vi "Motion_Profiling.vi"() -> ()   [LabVIEW 2015]
uses:
  <vilib>/Rock Robotics/WPI/Utilities/WPI_GetSetVariantRefNum.vi
panel:
  in  "Max Speed":dbl=120.0 format="%#_13g"
  in  "Max Accel":dbl=80.0 format="%#_13g"
  in  "Max Jerk":dbl=80.0 format="%#_13g"
  in  "forward":bool=TRUE
  in  "DistanceR (in)":dbl=180.0
  in  "DistanceL (in)":dbl=180.0
  in  "Auto Control":bool=TRUE
  in  "Constants":T1={"kV"=0.009, "kA"=0.0, "PV"=0.0, "PP"=0.0, "DV"=0.0}
  out "Position Chart":cluster{"pos":dbl, "pos":dbl, "pos":dbl}(graph)
  in  "Duty Cycle":dbl(slide)=0.015603286203016431 scale=-1.0..1.0
  out "Velocity Chart":cluster{"vel":dbl, dbl, "vel":dbl}(graph)
  in  "Chart Slowing":u32(knob)=4 scale=1.0..10.0
  # "Remember to make default!"
  # "backward"
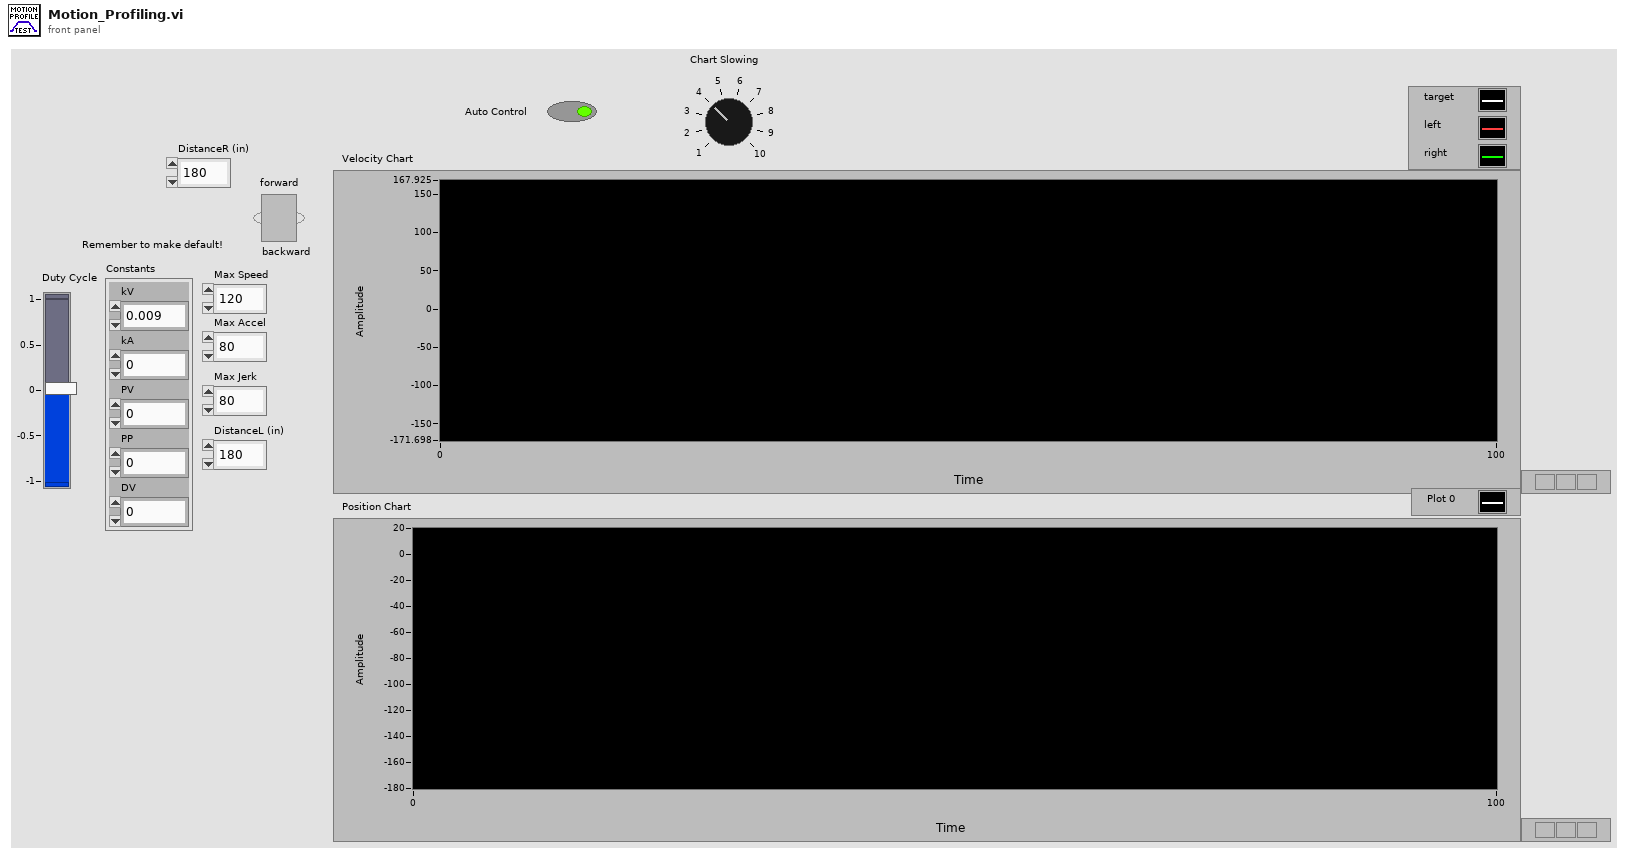
[diagram p1: front panel]
types:
  T1 = cluster{"kV":dbl, "kA":dbl, "PV":dbl, "PP":dbl, "DV":dbl}
  T2 = cluster{"Positions":dbl[], "Velocities":dbl[], "Accelerations":dbl[]}
  T3 = typedef "WPI_PotentiometerDevRef.ctl" = cluster{"DevStatus":errorcluster, "Analog Channel":T4, "Invert Output":bool}
  T4 = typedef "FPGA_AIChannel.ctl" = enum8{"AI 0", "AI 1", "AI 2", "AI 3", "AI MXP 0", "AI MXP 1", "AI MXP 2", "AI MXP 3", "Invalid"}
  T5 = typedef "WPI_RobotDriveDevRef.ctl" = cluster{"DevStatus":errorcluster, "Motors[]":T6[], "Square Inputs":bool, "Max Output":dbl}
  T6 = typedef "WPI_MotorControlDeviceRef.ctl" = cluster{"DeviceStatus":errorcluster, "Type":T7, "PWM":cluster{"PWM Channel":T8, "DeadBand":T9}, "CAN":cluster{"Device Number":u8, "Control Mode":T10, "Semaphore":T11, "Max Vout":dbl, "TalonSRX Control Mode":T12}, "Invert":bool}
  T7 = typedef "WPI_MotorControlType.ctl" = enum16{"PWM", "CAN", "CANTalonSRX"}
  T8 = typedef "FPGA_DIOPWMChannel.ctl" = enum8{"PWM 0", "PWM 1", "PWM 2", "PWM 3", "PWM 4", "PWM 5", "PWM 6", "PWM 7", "PWM 8", "PWM 9", "PWM MXP 0", "PWM MXP 1", "PWM MXP 2", "PWM MXP 3", "PWM MXP 4", "PWM MXP 5", "PWM MXP 6", "PWM MXP 7", "PWM MXP 8", "PWM MXP 9", "Invalid"}
  T9 = typedef "WPI_PWMDeadband.ctl" = cluster{"Name":string, "maxPositivePwm":i32, "minPositivePwm":i32, "centerPwm":i32, "maxNegativePwm":i32, "minNegativePwm":i32, "angularRange":u16}
  T10 = typedef "WPI_CANJaguar_ControlMode.ctl" = enum8{"Percent VBus", "Current", "Speed", "Position", "Voltage"}
  T11 = typedef "Semaphore RefNum" = refnum<k1>
  T12 = typedef "WPI_CANTalonSRX_APIControlMode.ctl" = enum8{"Percent VBus", "Speed", "Position", "Slave", "Unchanged / Invalid", "Voltage Compensation", "Current", "Motion Profile"}
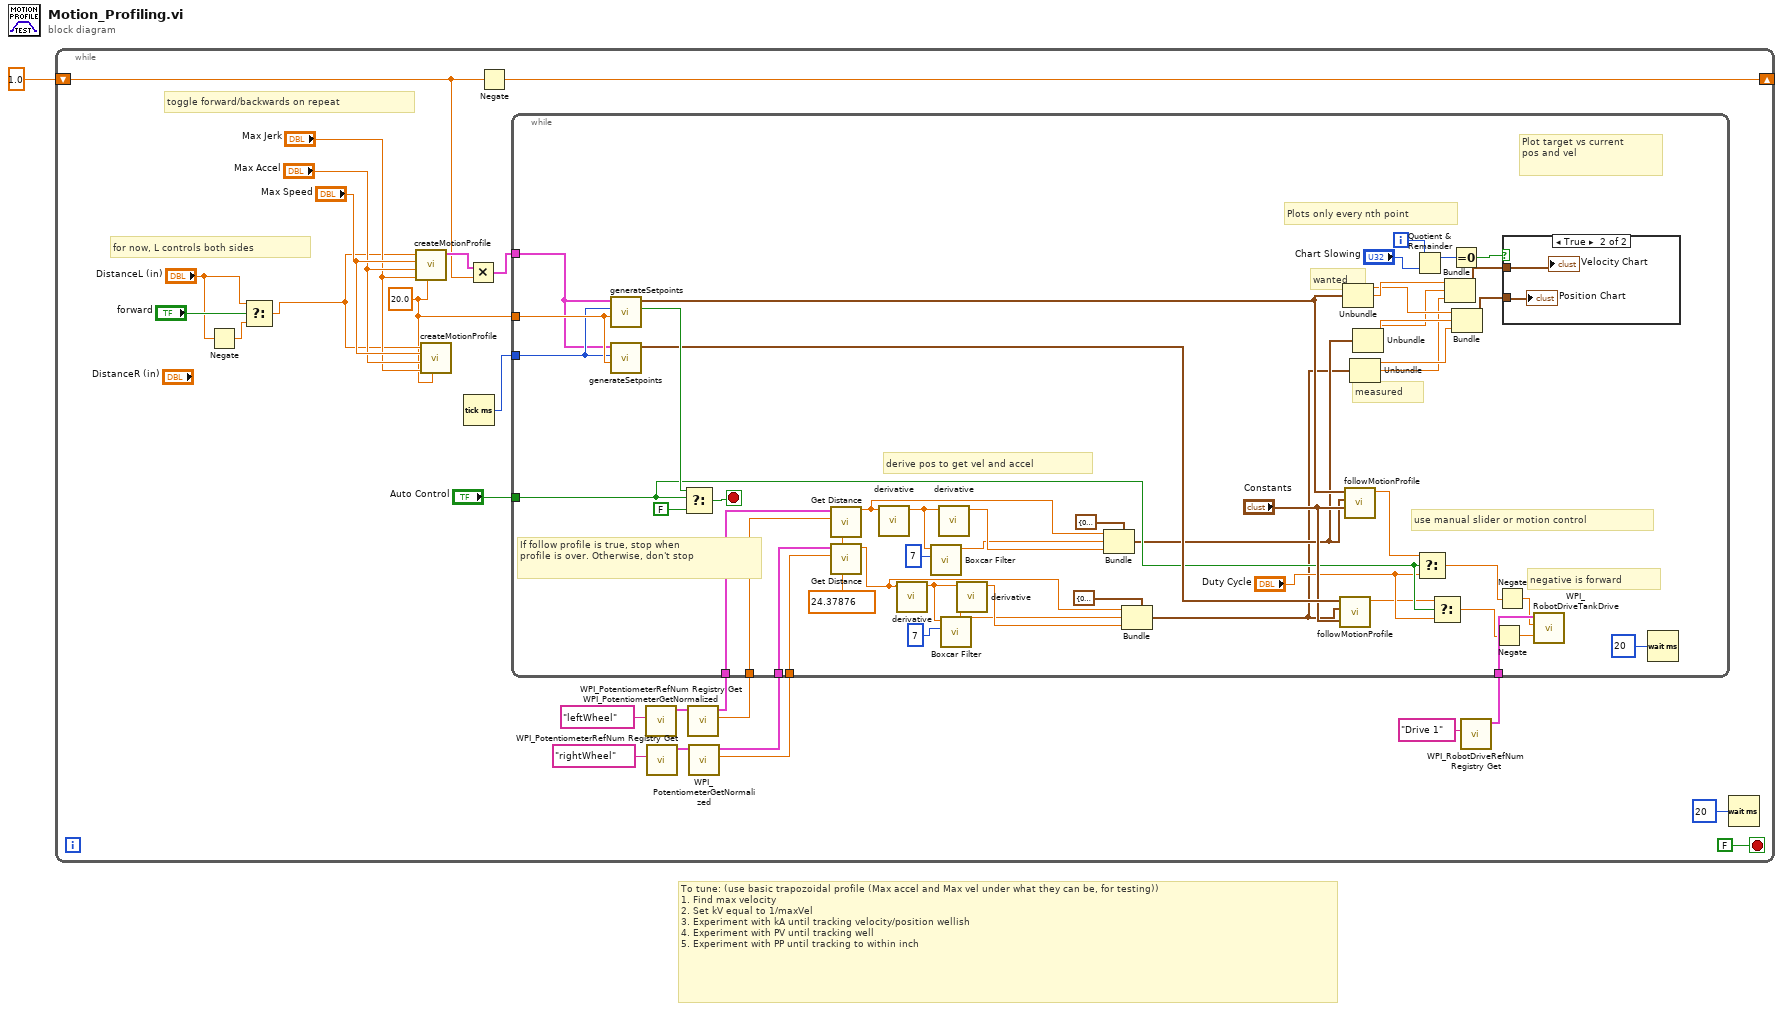
[diagram p0: block diagram]
diagram:
  # "To tune: (use basic trapozoidal profile (Max accel and Max vel under what they can be, for testing))\n1. Find max velocity\n2. Set kV equal to 1/maxVel\n3. Experiment with kA until tracking velocity/position wellish\n4. Experiment with PV until tracking well\n5. Experiment with PP until tracking to within inch"
  n1 = while {
    shift-right: [w4] -> _
    shift-left: 1.0 ("Motion Profile Control Frame Rate") -> [w6]
    stop <- FALSE stop-if-true
    w9 = 20.0 ("Motion Profile Control Frame Rate")
    # "toggle forward/backwards on repeat"
    # "for now, L controls both sides"
    n2 = Negate(x="DistanceL (in)") -> (-x=w12:dbl)
    n3 = Select(t="DistanceL (in)", s="forward", f=w12) -> (s? t:f=w10:dbl)
    n4 = call "createMotionProfile.vi"("ms per frame"=w9, "Max Jerk (In/sec^3)"="Max Jerk", "Max Acceleration (In/sec^2)"="Max Accel", "Max Speed (In/sec)"="Max Speed", "Inches to Travel"=w10) -> ("Profile"=w7:T2)  [unwired: 6 in]
    n5 = call "createMotionProfile.vi"("ms per frame"=w9, "Max Jerk (In/sec^3)"="Max Jerk", "Max Acceleration (In/sec^2)"="Max Accel", "Max Speed (In/sec)"="Max Speed", "Inches to Travel"=w10) -> ()  [unwired: 6 in, 1 out]
    n6 = Tick Count (ms)() -> (millisecond timer value=w8:u32)
    n7 = Multiply(x=w7, y=w6) -> (x*y=w5:T2)
    n8 = Negate(x=w6) -> (-x=w4:dbl)
    n9 = call <vilib>:"WPI_PotentiometerRefNum Registry Get.vi"("refnum name"="leftWheel") -> ("PotDevRef"=w24:T3)  [unwired: 9 in, 1 out]
    n10 = call <vilib>:"WPI_PotentiometerRefNum Registry Get.vi"("refnum name"="rightWheel") -> ("PotDevRef"=w23:T3)  [unwired: 9 in, 1 out]
    n11 = call <vilib>:"WPI_PotentiometerGetNormalized.vi"("PotDevRef"=w24) -> ("Normalized Value"=w17:dbl, "PotDevRef"=w20:T3)  [unwired: 8 in, 1 out]
    n12 = call <vilib>:"WPI_PotentiometerGetNormalized.vi"("PotDevRef"=w23) -> ("Normalized Value"=w18:dbl, "PotDevRef"=w19:T3)  [unwired: 8 in, 1 out]
    n13 = call <vilib>:"WPI_RobotDriveRefNum Registry Get.vi"("refnum name"="Drive 1") -> ("RobotDriveDevRef"=w25:T5)  [unwired: 9 in, 1 out]
    n14 = while {
      tunnel: "Auto Control" -> [w55]
      tunnel: w25 -> [w72]
      tunnel: w20 -> [w71]
      tunnel: w19 -> [w70]
      tunnel: w18 -> [w69]
      tunnel: w17 -> [w68]
      tunnel: w5 -> [w34]
      tunnel: w9 -> [w40]
      tunnel: w8 -> [w39]
      i -> [w77]
      stop <- w76 stop-if-true
      w67 = 24.37876 ("distance/rotation")
      # "negative is forward"
      # "wanted"
      # "measured"
      # "derive pos to get vel and accel"
      # "Plot target vs current\npos and vel"
      # "Plots only every nth point"
      # "use manual slider or motion control"
      # "If follow profile is true, stop when\nprofile is over. Otherwise, don't stop"
      n15 = call "generateSetpoints.vi"("ms/frame"=w40, "start time"=w39, "Profile"=w34) -> ("Done?"=w65:bool, "Setpoint"=w59:cluster{"pos":dbl, "vel":dbl, "accel":dbl})  [unwired: 7 in]
      n16 = call "generateSetpoints.vi"("ms/frame"=w40, "start time"=w39, "Profile"=w34) -> ("Setpoint"=w57:cluster{"pos":dbl, "vel":dbl, "accel":dbl})  [unwired: 7 in, 1 out]
      n17 = Select(t=w65, s=w55, f=FALSE) -> (s? t:f=w76:bool)
      n18 = call "Get Distance.vi"("distance/rotation"=w67, "Starting value"=w68, "PotDevRef"=w71) -> ("Distance"=w43:dbl)  [unwired: 8 in]
      n19 = call "Get Distance.vi"("distance/rotation"=w67, "Starting value"=w69, "PotDevRef"=w70) -> ("Distance"=w46:dbl)  [unwired: 8 in]
      n20 = call "derivative.vi"("x"=w43) -> ("dx/dt"=w33:dbl)  [unwired: 10 in]
      n21 = call "derivative.vi"("x"=w46) -> ("dx/dt"=w29:dbl)  [unwired: 10 in]
      n22 = call "Boxcar Filter.vi"("Points to average"=7, "Input"=w33) -> ("Average"=w31:dbl)  [unwired: 9 in]
      n23 = call "derivative.vi"("x"=w33) -> ("dx/dt"=w44:dbl)  [unwired: 10 in]
      n24 = call "Boxcar Filter.vi"("Points to average"=7, "Input"=w29) -> ("Average"=w28:dbl)  [unwired: 9 in]
      n25 = call "derivative.vi"("Starting value"=w28, "x"=w29) -> ("dx/dt"=w45:dbl)  [unwired: 9 in]
      n26 = Bundle(cluster=cluster{"pos":dbl, "vel":dbl, "accel":dbl} {"pos"=0.0, "vel"=0.0, "accel"=0.0}, "pos"=w43, "vel"=w31, "accel"=w44) -> (w48:cluster{"pos":dbl, "vel":dbl, "accel":dbl})
      n27 = Bundle(cluster=cluster{"pos":dbl, "vel":dbl, "accel":dbl} {"pos"=0.0, "vel"=0.0, "accel"=0.0}, "pos"=w46, "vel"=w28, "accel"=w45) -> (w38:cluster{"pos":dbl, "vel":dbl, "accel":dbl})
      n28 = call "followMotionProfile.vi"("Constants"="Constants", "Feedback"=w38, "Target"=w57) -> ("Duty Cycle"=w53:dbl)  [unwired: 8 in]
      n29 = Unbundle(w59) -> ("pos"=w42:dbl, "vel"=w58:dbl)  [unwired: 1 out]
      n30 = call "followMotionProfile.vi"("Constants"="Constants", "Feedback"=w48, "Target"=w59) -> ("Duty Cycle"=w73:dbl)  [unwired: 8 in]
      n31 = Unbundle(w38) -> ("pos"=w37:dbl, "vel"=w36:dbl)  [unwired: 1 out]
      n32 = Unbundle(w48) -> ("pos"=w41:dbl, "vel"=w35:dbl)  [unwired: 1 out]
      n33 = Quotient & Remainder(x=w77, y="Chart Slowing") -> (x-y*floor(x/y)=w64:u32)  [unwired: 1 out]
      n34 = Select(t=w73, s=w55, f="Duty Cycle") -> (s? t:f=w52:dbl)
      n35 = Select(t=w53, s=w55, f="Duty Cycle") -> (s? t:f=w49:dbl)
      n36 = Bundle("vel"=w58, "vel"=w35, "vel"=w36) -> (w60:cluster{"vel":dbl, "vel":dbl, "vel":dbl})  [unwired: 1 in]
      n37 = Equal To 0?(x=w64) -> (x = 0?=w63:bool)
      n38 = Bundle("pos"=w42, "pos"=w41, "pos"=w37) -> (w61:cluster{"pos":dbl, "pos":dbl, "pos":dbl})  [unwired: 1 in]
      n39 = Negate(x=w49) -> (-x=w50:dbl)
      n40 = Negate(x=w52) -> (-x=w51:dbl)
      n41 = case shown="True" w63 {
        tunnel: w61 -> [_ w79]
        tunnel: w60 -> [_ w78]
        frame False {
        }
        frame True {
          "Velocity Chart" <- w78
          "Position Chart" <- w79
        }
      }
      n42 = call <vilib>:"WPI_RobotDriveTankDrive.vi"("Right axis value"=w50, "Left axis value"=w51, "RobotDriveDevRef"=w72) -> ()  [unwired: 6 in, 3 out]
      n43 = Wait (ms)(milliseconds to wait=u32 20) -> ()  [unwired: 1 out]
    }
    n44 = Wait (ms)(milliseconds to wait=u32 20) -> ()  [unwired: 1 out]
  }
